vi "Blink 4 experimental.vi"(8 "Error In":errorcluster) -> (0 "Error Out":errorcluster)   [LabVIEW 2014]
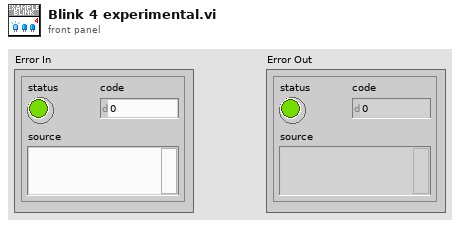
[diagram p1: front panel]
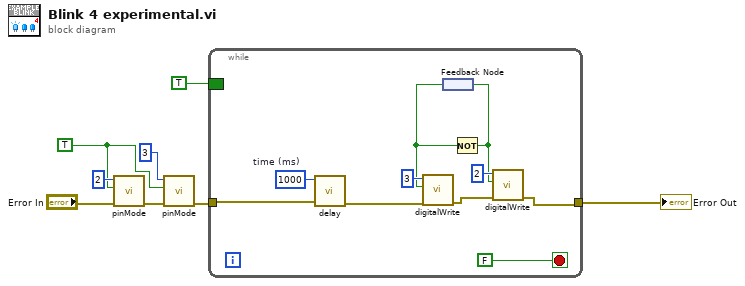
[diagram p0: block diagram]
diagram:
  w2 = TRUE
  n1 = call "pinMode.vi"("Error In"="Error In", "output?"=w2, "pin number"=2) -> ("Error Out"=w6:errorcluster)  [unwired: 8 in]
  n2 = call "pinMode.vi"("Error In"=w6, "output?"=w2, "pin number"=3) -> ("Error Out"=w7:errorcluster)  [unwired: 8 in]
  n3 = while {
    tunnel: w7 -> [w18]
    tunnel: [w15] -> w8
    border: TRUE -> [_]
    stop <- FALSE stop-if-true
    w16 = 1000  # time (ms)
    n4 = call "delay.vi"("Error In"=w18, "time (ms)"=w16) -> ("Error Out"=w17:errorcluster)  [unwired: 9 in]
    n5 = feedback #1() -> (w10:bool)
    n6 = call "digitalWrite.vi"("Error In"=w17, "value"=w10, "pin number"=3) -> ("Error Out"=w11:errorcluster)  [unwired: 8 in]
    n7 = Not(x=w10) -> (.not. x?=w9:bool)
    n8 = feedback-in #1(w9) -> ()
    n9 = call "digitalWrite.vi"("Error In"=w11, "value"=w9, "pin number"=2) -> ("Error Out"=w15:errorcluster)  [unwired: 8 in]
  }
  "Error Out" <- w8
